vi "Joint Reference Follower (beta).vi"(6 "Accurus Ctrl Cluster":T2={"Stop Vacuum"=TRUE, "Vacuum Force"=0, "Max Limit [mmHg]"=600.0, "Slide in"=0, "Irrigation?"=TRUE} {"Slide in" scale=0.0..78.0; "Vacuum Force" min=0 max=78}, 7 "Offset Home2RCM [deg/mm]":dbl[](array[numeric])=[0.0, 0.0, 0.0, 0.0], 8 "PID Ctrl Cluster":T3={"L1 PID Gains"={"Kp"=0.005, "Kd"=0.5, "Ki"=0.0005}, "L2 PID Gains"={"Kp"=0.01, "Kd"=1.0, "Ki"=0.005}, "L3 PID Gains"={"Kp"=0.05, "Kd"=1.0, "Ki"=0.0005}, "L4 PID Gains"={"Kp"=0.1, "Kd"=0.1, "Ki"=0.0005}}, 9 "Ref Array [deg/mm]":dbl[](array[numeric])=[0.0, 0.0, 0.0, 0.0], 10 "error in":errorcluster, 11 "FPGA VI Reference In":refnum<k20>) -> (0 "Accurus Output Cluster":T1, 1 "Output Posit Array [deg/mm]":dbl[](array[numeric]), 2 "error out":errorcluster, 3 "FPGA VI Reference Out":refnum<k20>)   [LabVIEW 2016]
uses:
  <vilib>/rvi/errors/niLvFpgaAdjustHostInterfaceError.vi
  <vilib>/Utility/error.llb/Error Cluster From Error Code.vi
  Subsystems/Global Variables.vi
  <vilib>/rvi/interface/nirviReadWriteControl/nirviReadWriteControl.xnode
  FPGA Bitfiles/IRISSTrack_FPGATarget2_IRISSFPGAIORIO_4NTO9ubhv-c.lvbitx
  IRISS_FPGA_IO_RIO.vi
  Library/KevinLibraryAll/labview/KevLib01.lvlib
  NiFpgaLv.dll
panel:
  # "button 1"
  # "button 2"
  # "button 3"
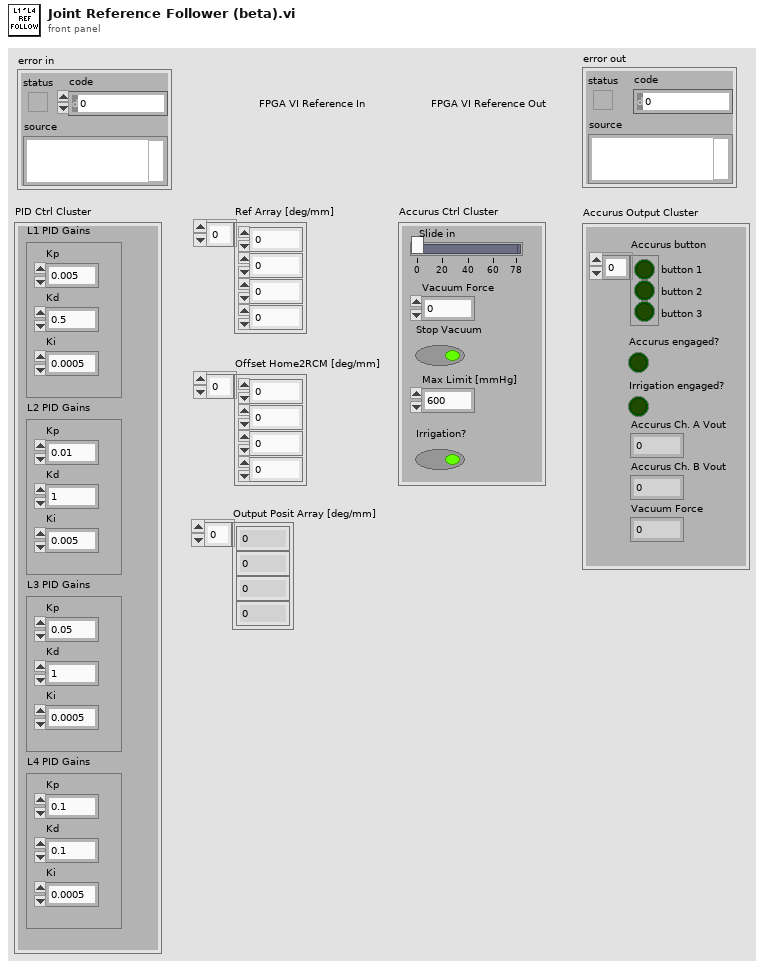
[diagram p1: front panel]
types:
  T1 = cluster{"Accurus button":bool[], "Accurus engaged?":bool, "Vacuum Force":i32, "Accurus Ch. A Vout":dbl, "Accurus Ch. B Vout":dbl, "Irrigation engaged?":bool}
  T2 = cluster{"Stop Vacuum":bool, "Vacuum Force":i8, "Max Limit [mmHg]":dbl, "Slide in":i8, "Irrigation?":bool}
  T3 = cluster{"L1 PID Gains":cluster{"Kp":dbl, "Kd":dbl, "Ki":dbl}, "L2 PID Gains":cluster{"Kp":dbl, "Kd":dbl, "Ki":dbl}, "L3 PID Gains":cluster{"Kp":dbl, "Kd":dbl, "Ki":dbl}, "L4 PID Gains":cluster{"Kp":dbl, "Kd":dbl, "Ki":dbl}}
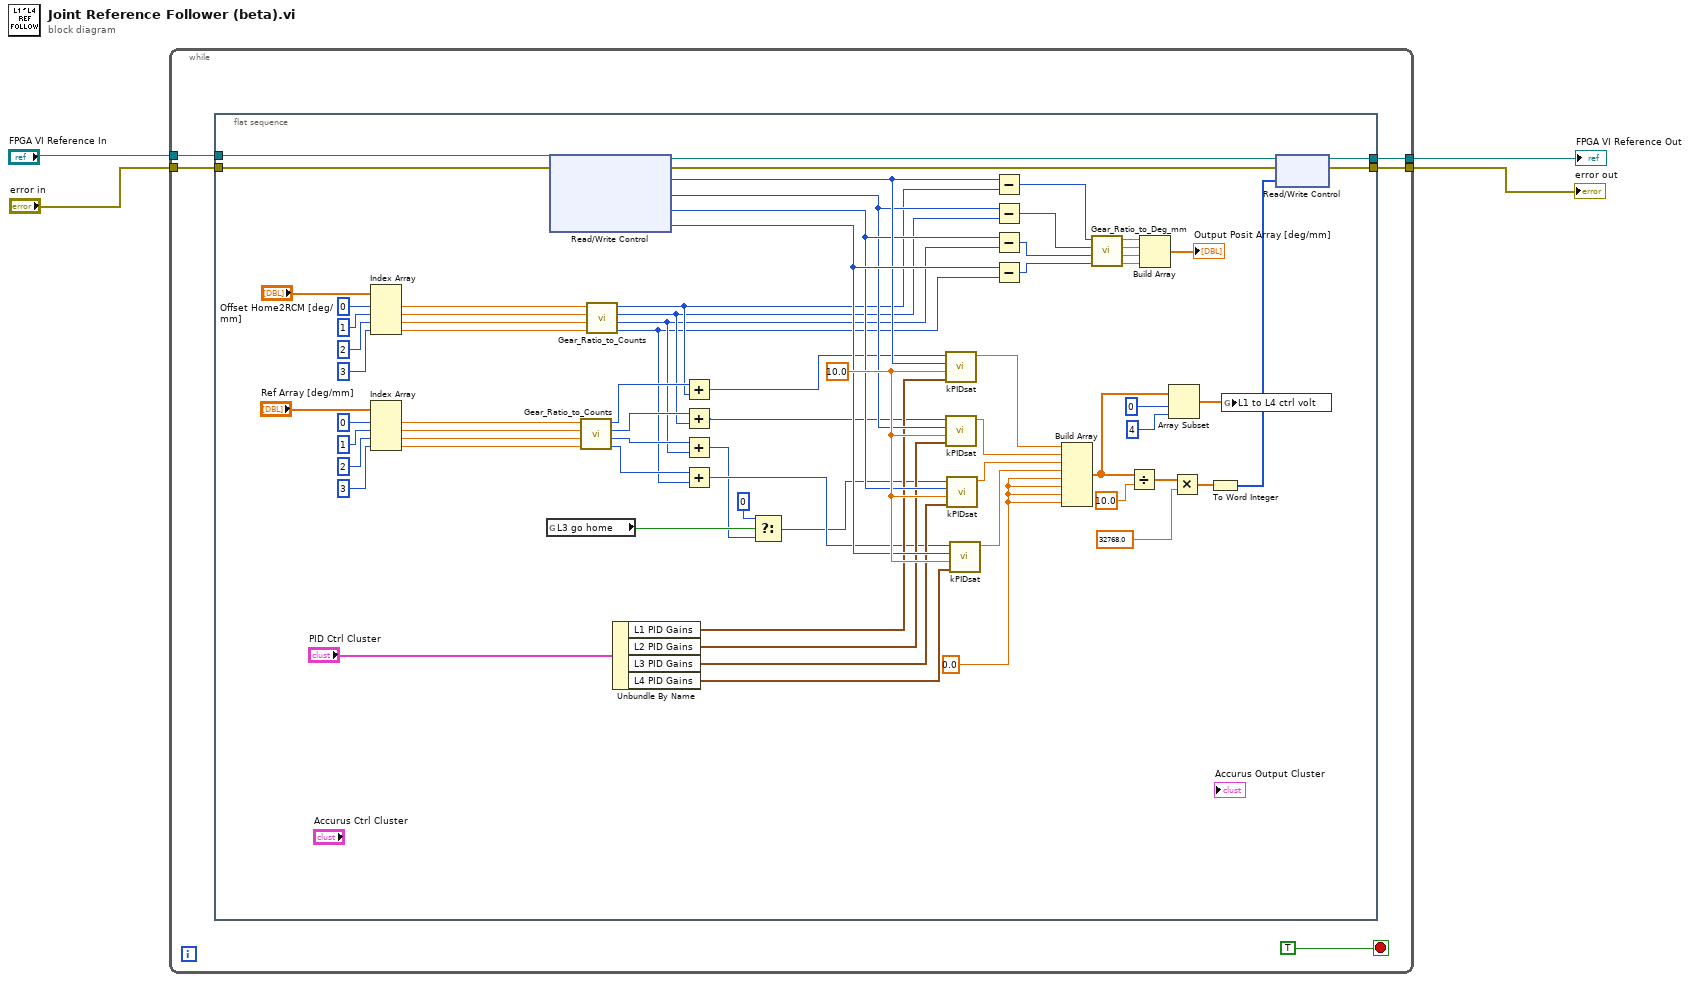
[diagram p0: block diagram]
diagram:
  n1 = while {
    tunnel: [w9] -> w1
    tunnel: [w8] -> w4
    tunnel: "FPGA VI Reference In" -> [w7]
    tunnel: "error in" -> [w6]
    stop <- TRUE ("Boolean") stop-if-true
    n2 = flat-sequence {
      tunnel: [w58] -> w9
      tunnel: [w57] -> w8
      tunnel: w7 -> [w36]
      tunnel: w6 -> [w35]
      frame #0 {
        w11 = 0.0 ("element")
        w67 = 10.0 ("Sat Limit")
        n3 = Index Array(array="Offset Home2RCM [deg/mm]", index #1=0 ("index"), index #2=1 ("index"), index #3=2 ("index"), index #4=3 ("index")) -> (element #1=w34:dbl, element #2=w33:dbl, element #3=w32:dbl, element #4=w31:dbl)
        n4 = Index Array(array="Ref Array [deg/mm]", index #1=0 ("index"), index #2=1 ("index"), index #3=2 ("index"), index #4=3 ("index")) -> (element #1=w75:dbl, element #2=w74:dbl, element #3=w73:dbl, element #4=w10:dbl)
        n5 = global read "Global Variables.vi" "L3 go home"() -> (w19:bool)
        n6 = xnode "Read/Write Control"("FPGA VI Reference In"=w36, "error in"=w35) -> ("FPGA VI Reference Out"=w60:refnum<k20>, "error out"=w59:errorcluster, "32 bit Position 1"=w43:i32, "32 bit Position 3"=w41:i32, "32 bit Position C1-1"=w42:i32, "32 bit Position C1-4"=w53:i32)
        n7 = call "Gear_Ratio_to_Counts.vi"("theta 4"=w10, "theta 3"=w73, "theta 2"=w74, "theta 1"=w75) -> ("j4"=w24:i32, "j3"=w25:i32, "j2"=w26:i32, "j1"=w27:i32)
        n8 = call "Gear_Ratio_to_Counts.vi"("theta 4"=w31, "theta 3"=w32, "theta 2"=w33, "theta 1"=w34) -> ("j4"=w20:i32, "j3"=w21:i32, "j2"=w22:i32, "j1"=w23:i32)
        n9 = Unbundle By Name("PID Ctrl Cluster") -> ("L1 PID Gains"=w40:cluster{"Kp":dbl, "Kd":dbl, "Ki":dbl}, "L2 PID Gains"=w39:cluster{"Kp":dbl, "Kd":dbl, "Ki":dbl}, "L3 PID Gains"=w38:cluster{"Kp":dbl, "Kd":dbl, "Ki":dbl}, "L4 PID Gains"=w37:cluster{"Kp":dbl, "Kd":dbl, "Ki":dbl})
        n10 = Add(x=w27, y=w23) -> (x+y=w30:i32)
        n11 = Add(x=w26, y=w22) -> (x+y=w29:i32)
        n12 = Add(x=w25, y=w21) -> (x+y=w18:i32)
        n13 = Add(x=w24, y=w20) -> (x+y=w28:i32)
        n14 = Select(t=0 ("index"), s=w19, f=w18) -> (s? t:f=w16:i32)
        n15 = call "kPIDsat.vi"("PID Gains"=w40, "Sat Limit"=w67, "Position"=w43, "Reference"=w30) -> ("Control"=w52:dbl)  [unwired: 7 in]
        n16 = call "kPIDsat.vi"("PID Gains"=w39, "Sat Limit"=w67, "Position"=w41, "Reference"=w29) -> ("Control"=w54:dbl)  [unwired: 7 in]
        n17 = call "kPIDsat.vi"("PID Gains"=w38, "Sat Limit"=w67, "Position"=w42, "Reference"=w16) -> ("Control"=w55:dbl)  [unwired: 7 in]
        n18 = call "kPIDsat.vi"("PID Gains"=w37, "Sat Limit"=w67, "Position"=w53, "Reference"=w28) -> ("Control"=w66:dbl)  [unwired: 7 in]
        n19 = Subtract(x=w43, y=w23) -> (x-y=w47:i32)
        n20 = Subtract(x=w41, y=w22) -> (x-y=w46:i32)
        n21 = Subtract(x=w42, y=w21) -> (x-y=w45:i32)
        n22 = Subtract(x=w53, y=w20) -> (x-y=w44:i32)
        n23 = Build Array(w52, w54, w55, w66, w11, w11, w11, w11) -> (w15:dbl[])
        n24 = call "Gear_Ratio_to_Deg_mm.vi"("j4"=w44, "j3"=w45, "j2"=w46, "j1"=w47) -> ("theta 4"=w48:dbl, "theta 3"=w49:dbl, "theta 2"=w50:dbl, "theta 1"=w51:dbl)
        n25 = Divide(x=w15, y=10.0) -> (x/y=w64:dbl[])
        n26 = Build Array(w51, w50, w49, w48) -> (→"Output Posit Array [deg/mm]":dbl[])
        n27 = Array Subset(array=w15, index=0, length=4) -> (w12:dbl[])
        n28 = Multiply(x=w64, y=32768.0) -> (x*y=w62:dbl[])
        n29 = To Word Integer(number=w62) -> (16bit integer=w61:i16[])
        n30 = global write "Global Variables.vi" "L1 to L4 ctrl volt"(w12) -> ()
        n31 = xnode "Read/Write Control"("FPGA VI Reference In"=w60, "error in"=w59, "AO"=w61) -> ("FPGA VI Reference Out"=w58:refnum<k20>, "error out"=w57:errorcluster)
      }
    }
  }
  "error out" <- w4
  "FPGA VI Reference Out" <- w1
